vi "set agc mode.vi"(8 "error in (no error)":errorcluster, 10 "on":bool, 11 "DevRefnum":u64) -> (0 "error out":errorcluster, 3 "DevRefnum":u64)   [LabVIEW 2013, in "rtlsdr.lvlib"]
doc: "RTLSDR_API int rtlsdr_set_agc_mode(rtlsdr_dev_t *dev, int on);"
uses:
  rtlsdr.lvlib
  rtlsdr.dll
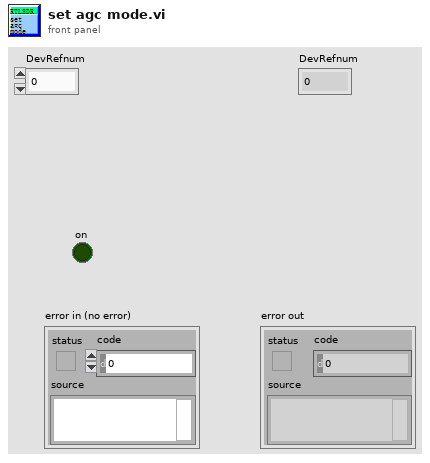
[diagram p1: front panel]
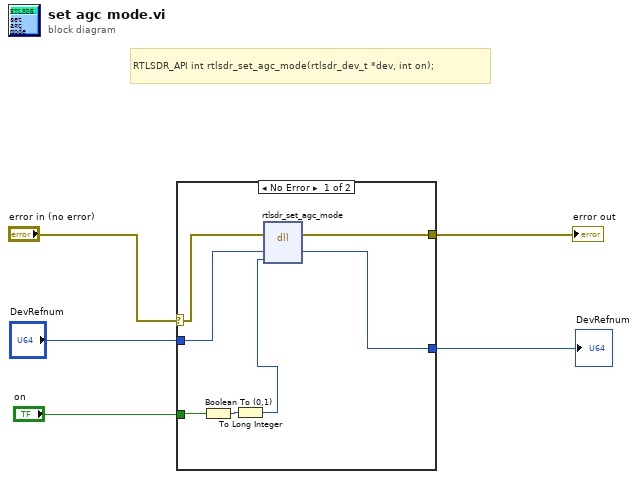
[diagram p0: block diagram]
diagram:
  # "RTLSDR_API int rtlsdr_set_agc_mode(rtlsdr_dev_t *dev, int on);"
  n1 = case shown="No Error" "error in (no error)" {
    selector: "error in (no error)" -> [w9 w14]
    tunnel: "on" -> [w8 _]
    tunnel: "DevRefnum" -> [w12 w13]
    tunnel: [w11 w13] -> w3
    tunnel: [w10 w14] -> w1
    frame No Error {
      n2 = Boolean To (0,1)(Boolean=w8) -> (0, 1=w7:i16)
      n3 = To Long Integer(number=w7) -> (32bit integer=w6:i32)
      n4 = dll-call lib="D:/SDRDriver/Lab1/rtlsdr.*" fn="rtlsdr_set_agc_mode"(error in=w9, "DevRefnum"=w12, "on"=w6) -> (error out=w10:errorcluster, "DevRefnum"=w11:u64)  [unwired: 4 in, 1 out]
    }
    frame Error {
    }
  }
  "error out" <- w1
  "DevRefnum" <- w3
